vi "Close Engine.vi"(8 "error in (no error)":errorcluster, 11 "Engine in":refnum<class "Engine.lvclass">) -> (0 "error out":errorcluster)   [LabVIEW 2020, in "TSnax.lvlib" / "Engine.lvclass"]
uses:
  Engine.lvclass
  Engine.lvclass/Engine.ctl
  Execution/Execution.lvclass
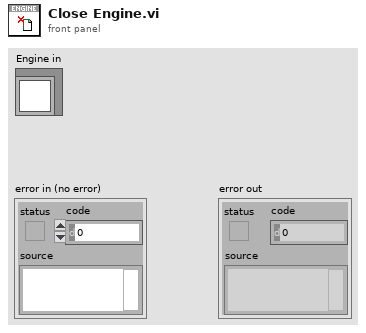
[diagram p1: front panel]
types:
  T1 = typedef "TSnax.lvlib/Engine.lvclass/Ref Data.ctl" = cluster{"Station Globals":refnum<class "PropertyObject.lvclass">, "Station Model":refnum<class "SequenceFile.lvclass">, "Trace Delay":u32, "Execution Map":map{i32, refnum<class "Execution.lvclass">}}
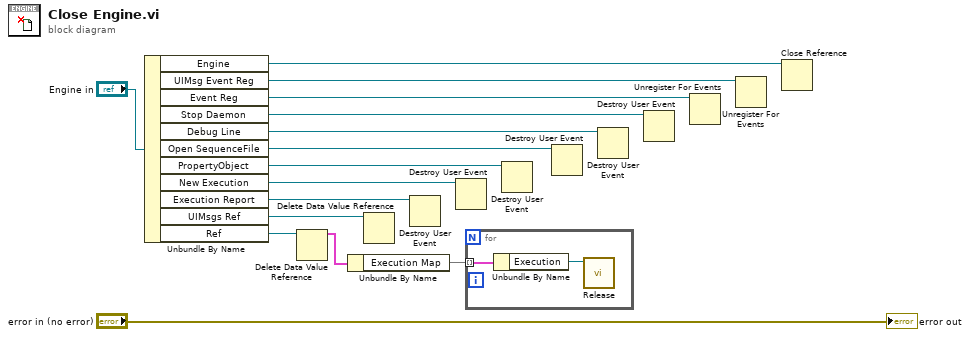
[diagram p0: block diagram]
diagram:
  n1 = Unbundle By Name("Engine in") -> ("Engine"=w10:refnum<k7>, "UIMsg Event Reg"=w11:refnum<k27>, "Event Reg"=w12:refnum<event-registration>, "Stop Daemon"=w13:refnum<user-event>, "Debug Line"=w9:refnum<user-event>, "Open SequenceFile"=w7:refnum<user-event>, "PropertyObject"=w5:refnum<user-event>, "New Execution"=w6:refnum<user-event>, "Execution Report"=w8:refnum<user-event>, "UIMsgs Ref"=w4:refnum<data-value>, "Ref"=w3:refnum<data-value>)
  n2 = Delete Data Value Reference(data value reference=w3) -> (data value=w2:T1)  [unwired: 1 in, 1 out]
  n3 = Unbundle By Name(w2) -> ("Execution Map"=w1:map{i32, refnum<class "Execution.lvclass">})
  n4 = Delete Data Value Reference(data value reference=w4) -> ()  [unwired: 1 in, 2 out]
  n5 = Destroy User Event(user event=w8) -> ()  [unwired: 1 in, 1 out]
  n6 = Destroy User Event(user event=w6) -> ()  [unwired: 1 in, 1 out]
  n7 = for {
    tunnel: w1 -> [w17] mode=indexing
    n8 = Unbundle By Name(w17) -> ("Execution"=w16:refnum<class "Execution.lvclass">)
    n9 = call-dynamic "Release.vi"("Execution in"=w16) -> ()  [unwired: 10 in, 1 out]
  }
  n10 = Destroy User Event(user event=w5) -> ()  [unwired: 1 in, 1 out]
  n11 = Destroy User Event(user event=w7) -> ()  [unwired: 1 in, 1 out]
  n12 = Destroy User Event(user event=w9) -> ()  [unwired: 1 in, 1 out]
  n13 = Destroy User Event(user event=w13) -> ()  [unwired: 1 in, 1 out]
  n14 = Unregister For Events(event registration refnum=w12) -> ()  [unwired: 1 in, 1 out]
  n15 = Unregister For Events(event registration refnum=w11) -> ()  [unwired: 1 in, 1 out]
  n16 = Close Reference(reference=w10) -> ()  [unwired: 1 in, 1 out]
  "error out" <- "error in (no error)"
